vi "Agilent N6700 Series Configure Voltage.vi"() -> ()   [LabVIEW 2021]
doc: "Configures the power supply's output range on a channel, configures the DC voltage level, channel appears at the output connector and takes a measurement on the output signal and returns the measured value."
uses:
  <instrlib>/Agilent 3446X Series/Public/Data/Read (Single Point).vi
  <instrlib>/Agilent N6700 Series/Agilent N6700 Series.lvlib
  <instrlib>/Agilent 3446X Series/Agilent 3446X Series.lvlib
panel:
  out "DMM Measurement":dbl
  in  "Manual Range (1)":dbl=1.0
  in  "Agilent DMM":refnum<visa-resource-name>
  in  "Absolute Resolution":dbl=1e-06
  in  "Measurement Function":i32(ring)=10 items=["Continuity", "Current AC", "Current DC", "Diode", "Frequency", "Resistance 4-wire", "Period", "Resistance 2-wire", "Temperature", "Voltage AC", "Voltage DC", "Voltage DC Ratio", "Capacitance"]
  in  "Vin SMU":refnum<visa-resource-name>
  in  "Vin SMUChannel":string="1"
  in  "Vin Voltage Range":dbl=10.0 format="%^.3e"
  in  "Vin Voltage Level":dbl=5.0 format="%^.3e"
  out "Vin Voltage Measurement":dbl format="%^.3e"
  in  "Vin Behavior":i32(ring) items=["Regulatory Limit", "Trip Limit"]
  in  "Vin Current Limit":dbl=1.0 format="%^.3e"
  in  "error in":errorcluster {"code" format="%.0x"}
  out "error out":errorcluster {"code" format="%.0x"}
  in  "Load Current Limit":dbl=1.0 format="%^.3e"
  in  "Load Behavior":i32(ring) items=["Regulatory Limit", "Trip Limit"]
  out "Load Voltage Measurement":dbl format="%^.3e"
  in  "Load Voltage Level":dbl=5.0 format="%^.3e"
  in  "Load Voltage Range":dbl=10.0 format="%^.3e"
  in  "Load SMUChannel":string="1"
  in  "Load SMU":refnum<visa-resource-name>
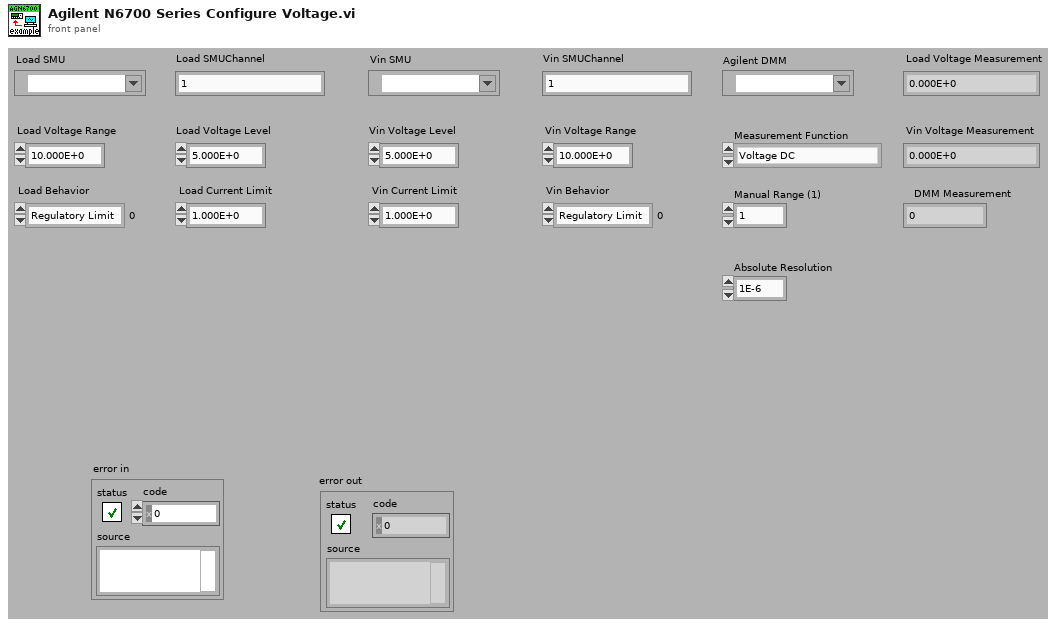
[diagram p1: front panel]
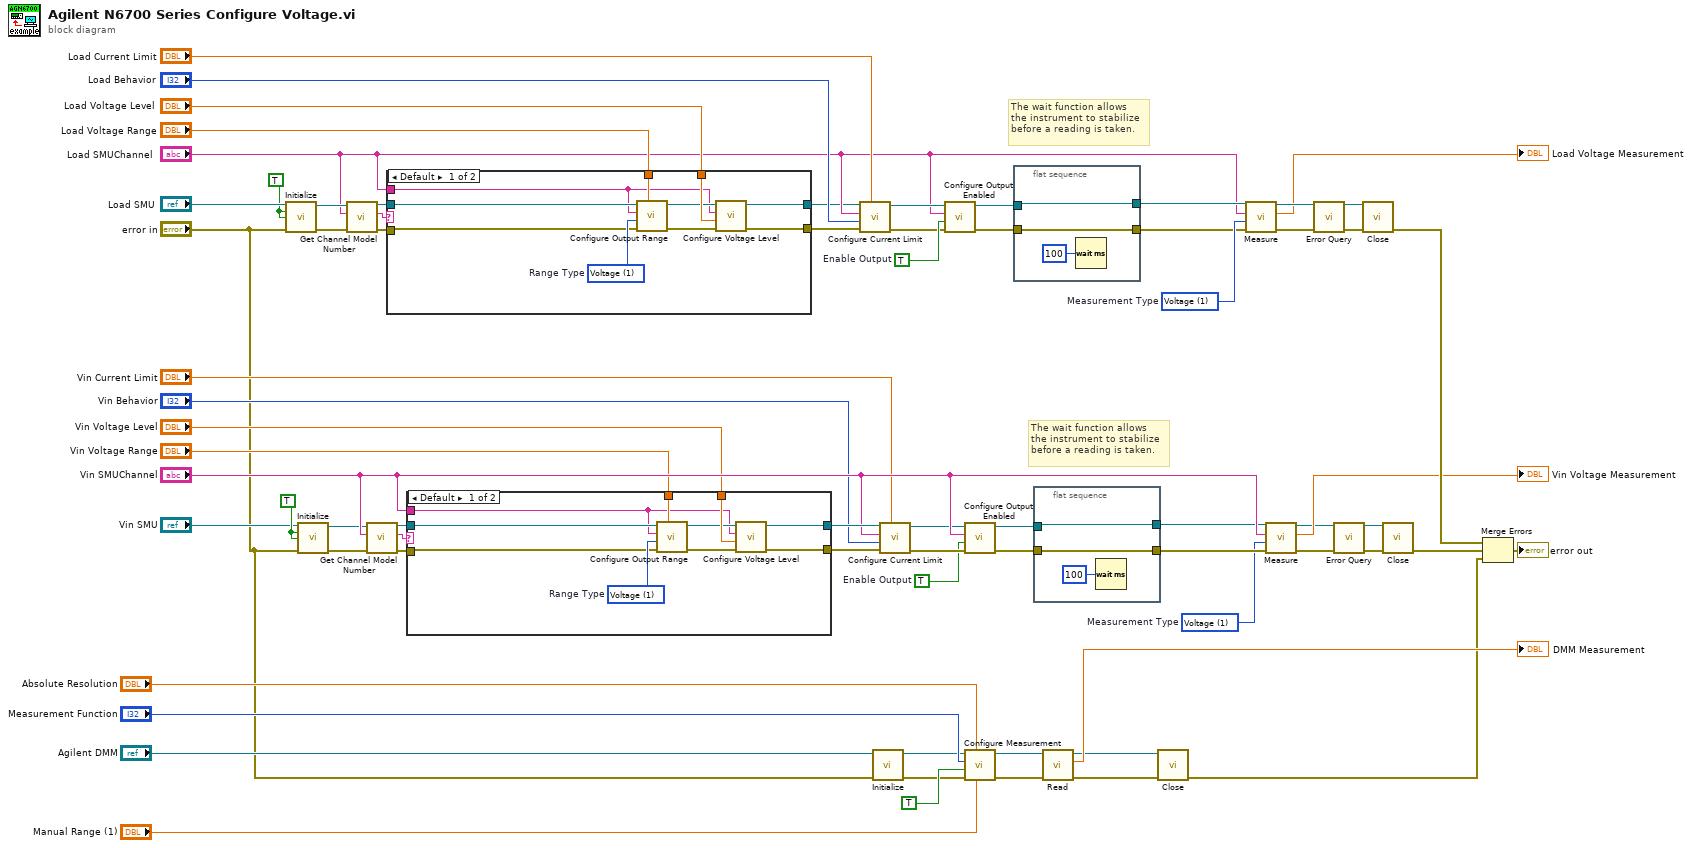
[diagram p0: block diagram]
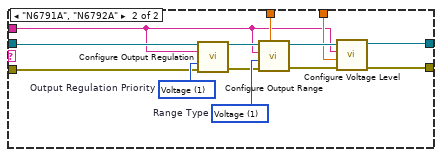
[diagram p2: hidden frame]
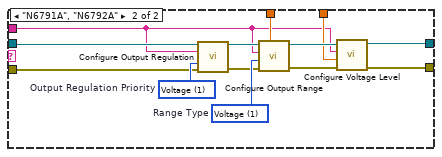
[diagram p3: hidden frame]
diagram:
  w26 = TRUE ("Reset? (T: Yes)")
  w25 = 1 items=["Voltage"=1, "Current"=0]  # Measurement Type
  w24 = TRUE  # Enable Output
  w62 = TRUE ("Reset? (T: Yes)")
  w63 = 1 items=["Voltage"=1, "Current"=0]  # Measurement Type
  w64 = TRUE  # Enable Output
  # "The wait function allows \nthe instrument to stabilize\nbefore a reading is taken."
  # "The wait function allows \nthe instrument to stabilize\nbefore a reading is taken."
  n1 = call <instrlib>:"Initialize.vi"("VISA resource name"="Load SMU", "ID Query? (T: Yes)"=w62, "Reset? (T: Yes)"=w62, "error in (no error)"="error in") -> ("VISA resource name out"=w53:refnum<visa-resource-name>, "error out"=w52:errorcluster)  [unwired: 10 in]
  n2 = call <instrlib>:"Initialize.vi"("VISA resource name"="Vin SMU", "ID Query? (T: Yes)"=w26, "Reset? (T: Yes)"=w26, "error in (no error)"="error in") -> ("VISA resource name out"=w35:refnum<visa-resource-name>, "error out"=w36:errorcluster)  [unwired: 10 in]
  n3 = call <instrlib>:"Get Channel Model Number.vi"("error in (no error)"=w52, "Channel Name (1)"="Load SMUChannel", "VISA resource name"=w53) -> ("error out"=w50:errorcluster, "Model Number"=w49:string, "VISA resource name out"=w51:refnum<visa-resource-name>)  [unwired: 6 in]
  n4 = call <instrlib>:"Get Channel Model Number.vi"("error in (no error)"=w36, "Channel Name (1)"="Vin SMUChannel", "VISA resource name"=w35) -> ("error out"=w38:errorcluster, "Model Number"=w39:string, "VISA resource name out"=w37:refnum<visa-resource-name>)  [unwired: 6 in]
  n5 = case shown="Default" w49 {
    tunnel: "Load Voltage Range" -> [w78 w94]
    tunnel: "Load SMUChannel" -> [w72 w84]
    tunnel: w51 -> [w80 w89]
    tunnel: w50 -> [w79 w88]
    tunnel: "Load Voltage Level" -> [w76 w85]
    tunnel: [w74 w82] -> w46
    tunnel: [w73 w83] -> w45
    frame Default {
      w81 = 1 items=["Voltage"=1, "Current"=0]  # Range Type
      n6 = call <instrlib>:"Configure Output Range.vi"("Range (0.0)"=w78, "error in (no error)"=w79, "Range Type (1: Voltage)"=w81, "Channel Name (1)"=w72, "VISA resource name"=w80) -> ("error out"=w77:errorcluster, "VISA resource name out"=w75:refnum<visa-resource-name>)  [unwired: 5 in]
      n7 = call <instrlib>:"Configure Voltage Level.vi"("error in (no error)"=w77, "Level  (0.0 volts)"=w76, "Channel Name (1)"=w72, "VISA resource name"=w75) -> ("error out"=w74:errorcluster, "VISA resource name out"=w73:refnum<visa-resource-name>)  [unwired: 6 in]
    }
    frame "N6791A", "N6792A" {
      w90 = 1 items=["Voltage"=1, "Current"=0]  # Output Regulation Priority
      w93 = 1 items=["Voltage"=1, "Current"=0]  # Range Type
      n8 = call <instrlib>:"Configure Output Regulation.vi"("VISA resource name"=w89, "Channel Name (1)"=w84, "Output Regulation Priority (1: Voltage)"=w90, "error in (no error)"=w88) -> ("VISA resource name out"=w92:refnum<visa-resource-name>, "error out"=w91:errorcluster)  [unwired: 10 in]
      n9 = call <instrlib>:"Configure Output Range.vi"("Range (0.0)"=w94, "error in (no error)"=w91, "Range Type (1: Voltage)"=w93, "Channel Name (1)"=w84, "VISA resource name"=w92) -> ("error out"=w86:errorcluster, "VISA resource name out"=w87:refnum<visa-resource-name>)  [unwired: 5 in]
      n10 = call <instrlib>:"Configure Voltage Level.vi"("error in (no error)"=w86, "Level  (0.0 volts)"=w85, "Channel Name (1)"=w84, "VISA resource name"=w87) -> ("error out"=w82:errorcluster, "VISA resource name out"=w83:refnum<visa-resource-name>)  [unwired: 6 in]
    }
  }
  n11 = case shown="Default" w39 {
    tunnel: "Vin Voltage Range" -> [w101 w117]
    tunnel: "Vin SMUChannel" -> [w95 w107]
    tunnel: w37 -> [w103 w112]
    tunnel: w38 -> [w102 w111]
    tunnel: "Vin Voltage Level" -> [w99 w108]
    tunnel: [w97 w105] -> w42
    tunnel: [w96 w106] -> w43
    frame Default {
      w104 = 1 items=["Voltage"=1, "Current"=0]  # Range Type
      n12 = call <instrlib>:"Configure Output Range.vi"("Range (0.0)"=w101, "error in (no error)"=w102, "Range Type (1: Voltage)"=w104, "Channel Name (1)"=w95, "VISA resource name"=w103) -> ("error out"=w100:errorcluster, "VISA resource name out"=w98:refnum<visa-resource-name>)  [unwired: 5 in]
      n13 = call <instrlib>:"Configure Voltage Level.vi"("error in (no error)"=w100, "Level  (0.0 volts)"=w99, "Channel Name (1)"=w95, "VISA resource name"=w98) -> ("error out"=w97:errorcluster, "VISA resource name out"=w96:refnum<visa-resource-name>)  [unwired: 6 in]
    }
    frame "N6791A", "N6792A" {
      w113 = 1 items=["Voltage"=1, "Current"=0]  # Output Regulation Priority
      w116 = 1 items=["Voltage"=1, "Current"=0]  # Range Type
      n14 = call <instrlib>:"Configure Output Regulation.vi"("VISA resource name"=w112, "Channel Name (1)"=w107, "Output Regulation Priority (1: Voltage)"=w113, "error in (no error)"=w111) -> ("VISA resource name out"=w115:refnum<visa-resource-name>, "error out"=w114:errorcluster)  [unwired: 10 in]
      n15 = call <instrlib>:"Configure Output Range.vi"("Range (0.0)"=w117, "error in (no error)"=w114, "Range Type (1: Voltage)"=w116, "Channel Name (1)"=w107, "VISA resource name"=w115) -> ("error out"=w109:errorcluster, "VISA resource name out"=w110:refnum<visa-resource-name>)  [unwired: 5 in]
      n16 = call <instrlib>:"Configure Voltage Level.vi"("error in (no error)"=w109, "Level  (0.0 volts)"=w108, "Channel Name (1)"=w107, "VISA resource name"=w110) -> ("error out"=w105:errorcluster, "VISA resource name out"=w106:refnum<visa-resource-name>)  [unwired: 6 in]
    }
  }
  n17 = call <instrlib>:"Configure Current Limit.vi"("Limit (0.0 amps)"="Load Current Limit", "error in (no error)"=w46, "Behavior (0: Regulatory Limit)"="Load Behavior", "Channel Name (1)"="Load SMUChannel", "VISA resource name"=w45) -> ("error out"=w61:errorcluster, "VISA resource name out"=w60:refnum<visa-resource-name>)  [unwired: 5 in]
  n18 = call <instrlib>:"Initialize.vi"("error in (no error)"="error in", "VISA resource name"="Agilent DMM") -> ("error out"=w6:errorcluster, "VISA resource name out"=w5:refnum<visa-resource-name>)  [unwired: 3 in, 5 out]
  n19 = call <instrlib>:"Configure Current Limit.vi"("Limit (0.0 amps)"="Vin Current Limit", "error in (no error)"=w42, "Behavior (0: Regulatory Limit)"="Vin Behavior", "Channel Name (1)"="Vin SMUChannel", "VISA resource name"=w43) -> ("error out"=w27:errorcluster, "VISA resource name out"=w28:refnum<visa-resource-name>)  [unwired: 5 in]
  n20 = call <instrlib>:"Configure Output Enabled.vi"("error in (no error)"=w61, "Enable Output (False)"=w64, "Channel Name (1)"="Load SMUChannel", "VISA resource name"=w60) -> ("error out"=w54:errorcluster, "VISA resource name out"=w57:refnum<visa-resource-name>)  [unwired: 6 in]
  n21 = call <instrlib>:"Configure Output Enabled.vi"("error in (no error)"=w27, "Enable Output (False)"=w24, "Channel Name (1)"="Vin SMUChannel", "VISA resource name"=w28) -> ("error out"=w34:errorcluster, "VISA resource name out"=w31:refnum<visa-resource-name>)  [unwired: 6 in]
  n22 = call <instrlib>:"Configure Measurement.vi"("Manual Range (1)"="Manual Range (1)", "Absolute Resolution (1E-6)"="Absolute Resolution", "error in (no error)"=w6, "Auto Range (T: Enable)"=TRUE, "Measurement Function (10: Voltage DC)"="Measurement Function", "VISA resource name"=w5) -> ("error out"=w8:errorcluster, "VISA resource name out"=w7:refnum<visa-resource-name>)  [unwired: 4 out]
  n23 = flat-sequence {
    tunnel: w57 -> [w120]
    tunnel: [w120] -> w56
    tunnel: [w118] -> w55
    tunnel: w54 -> [w118]
    frame #0 {
      n24 = Wait (ms)(milliseconds to wait=u32 100) -> ()  [unwired: 1 out]
    }
  }
  n25 = flat-sequence {
    tunnel: w31 -> [w123]
    tunnel: [w123] -> w32
    tunnel: [w121] -> w33
    tunnel: w34 -> [w121]
    frame #0 {
      n26 = Wait (ms)(milliseconds to wait=u32 100) -> ()  [unwired: 1 out]
    }
  }
  n27 = call-poly <instrlib>:"Read.vi"("error in (no error)"=w8, "VISA resource name"=w7) -> ("error out"=w2:errorcluster, "Measurement"=→"DMM Measurement":dbl, "VISA resource name out"=w3:refnum<visa-resource-name>)  [unwired: 7 out]
  n28 = call <instrlib>:"Close.vi"("error in (no error)"=w2, "VISA resource name"=w3) -> ("error out"=w1:errorcluster)  [unwired: 9 out]
  n29 = call <instrlib>:"Measure.vi"("error in (no error)"=w55, "Measurement Type (1: Voltage)"=w63, "Channel Name (1)"="Load SMUChannel", "VISA resource name"=w56) -> ("error out"=w71:errorcluster, "Measurement"=→"Load Voltage Measurement":dbl, "VISA resource name out"=w68:refnum<visa-resource-name>)  [unwired: 5 in]
  n30 = call <instrlib>:"Measure.vi"("error in (no error)"=w33, "Measurement Type (1: Voltage)"=w25, "Channel Name (1)"="Vin SMUChannel", "VISA resource name"=w32) -> ("error out"=w17:errorcluster, "Measurement"=→"Vin Voltage Measurement":dbl, "VISA resource name out"=w20:refnum<visa-resource-name>)  [unwired: 5 in]
  n31 = call <instrlib>:"Error Query.vi"("VISA resource name"=w68, "error in (no error)"=w71) -> ("VISA resource name out"=w69:refnum<visa-resource-name>, "error out"=w70:errorcluster)  [unwired: 10 in, 2 out]
  n32 = call <instrlib>:"Error Query.vi"("VISA resource name"=w20, "error in (no error)"=w17) -> ("VISA resource name out"=w19:refnum<visa-resource-name>, "error out"=w18:errorcluster)  [unwired: 10 in, 2 out]
  n33 = call <instrlib>:"Close.vi"("VISA resource name"=w69, "error in (no error)"=w70) -> ("error out"=w44:errorcluster)  [unwired: 13 in]
  n34 = call <instrlib>:"Close.vi"("VISA resource name"=w19, "error in (no error)"=w18) -> ("error out"=w15:errorcluster)  [unwired: 13 in]
  n35 = Merge Errors(w44, w15, w1) -> (→"error out":errorcluster)
